vi "MessagingPlayground.vi"() -> ()   [LabVIEW 2019]
uses:
  <userlib>/LevyLab/Instrument Framework/SMOs/RemoteControl/Typedefs/RC Com Type--enum.ctl
  <userlib>/LevyLab/Instrument Framework/SMOs/RemoteControl/RemoteControl.lvclass
  C:/Program Files (x86)/National Instruments/LabVIEW 2019/vi.lib/JKI/JKI SMO/SMO/SMO.lvclass
  <vilib>/JKI/JKI SMO/SMO/SMO.lvclass
panel:
  out "IDs":string[](array[string])
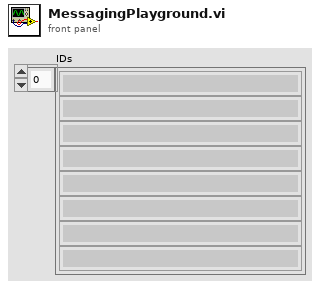
[diagram p1: front panel]
types:
  T1 = typedef "RemoteControl.lvclass/RC Com Type--enum.ctl" = enum16{"RC", "STM", "ZMQ"}
  T2 = enum32{"Invalid", "Standard", "Closed", "Hidden", "Minimized", "Maximized"}
  T3 = enum32{"invalid app kind", "Development System", "Run Time System", "Student Edition", "Embedded LabVIEW", "Evaluation", "Custom"}
  T4 = cluster{"Core":cluster{"Current VI Reference":refnum<vi>, "Close Panel on Exit?":bool}, "RC":refnum<class "RemoteControl.lvclass">, "IDs":string[]}
  T5 = cluster{"Current VI Reference":refnum<vi>, "Close Panel on Exit?":bool}
  T6 = typedef "RemoteControl.lvclass/PublicEvents--Cluster.ctl" = cluster{"SendMessageFromProcess":refnum<user-event>}
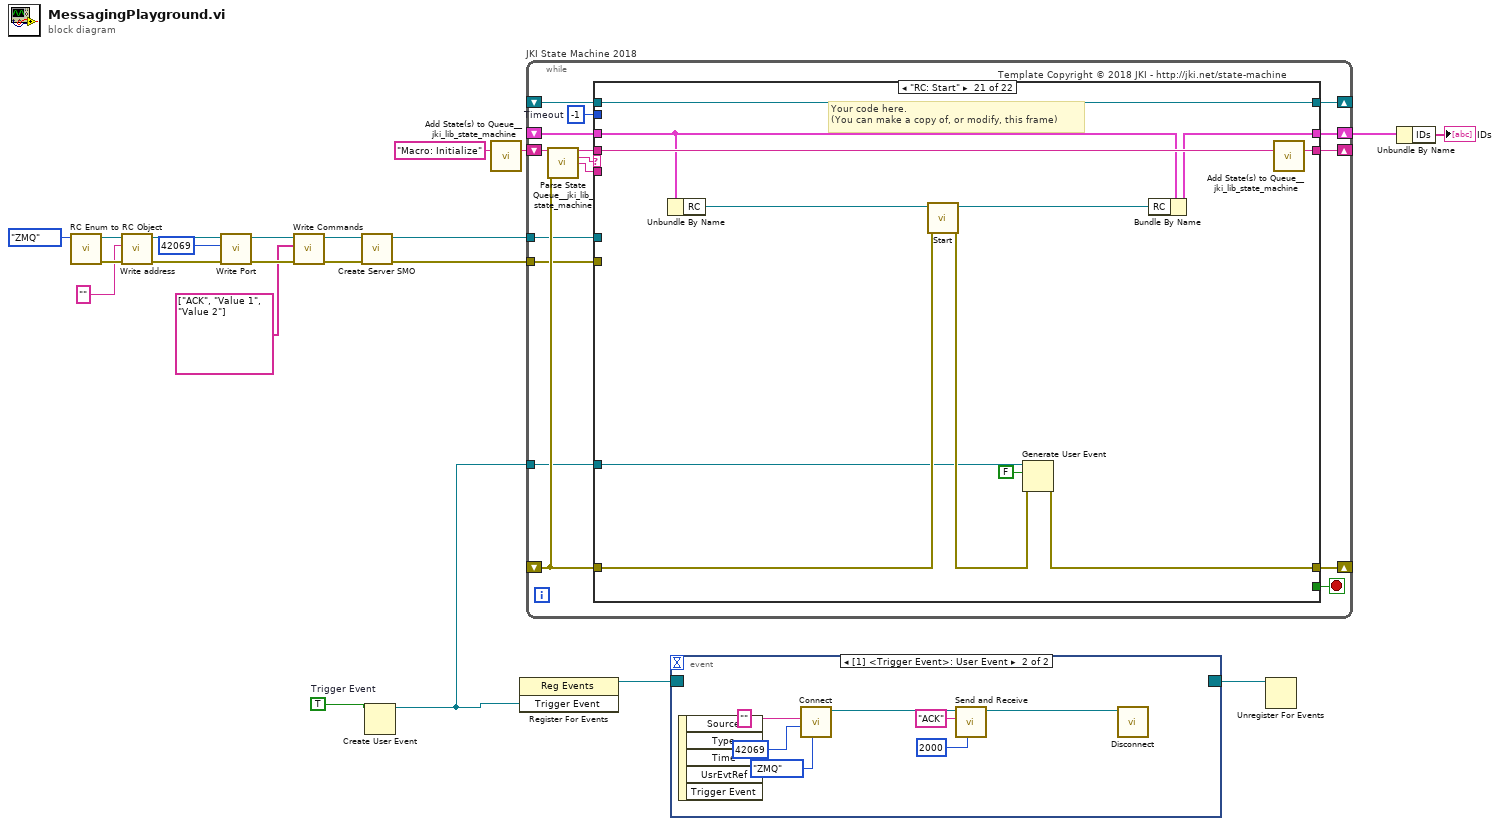
[diagram p0: block diagram]
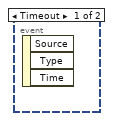
[diagram p2: hidden frame]
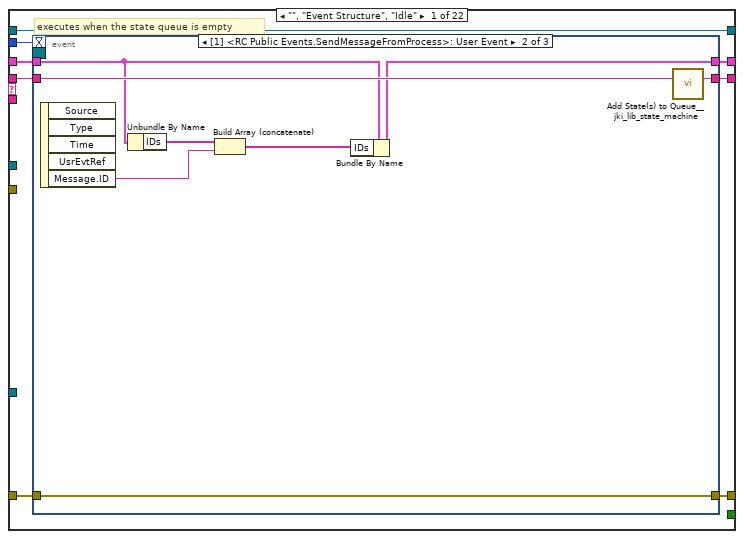
[diagram p3: hidden frame]
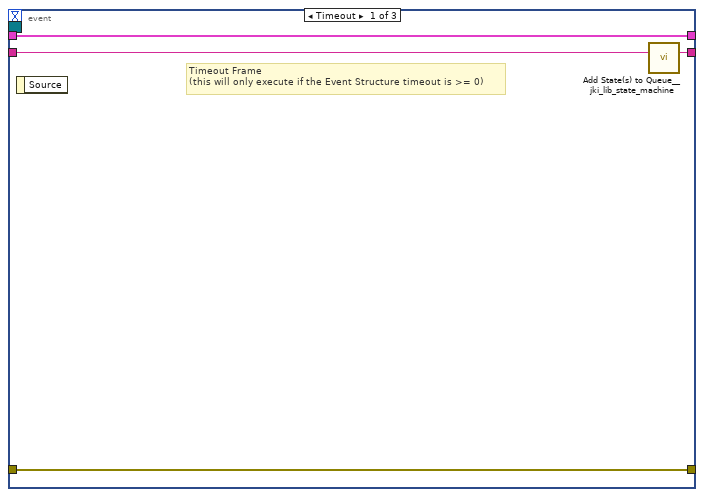
[diagram p4: hidden frame]
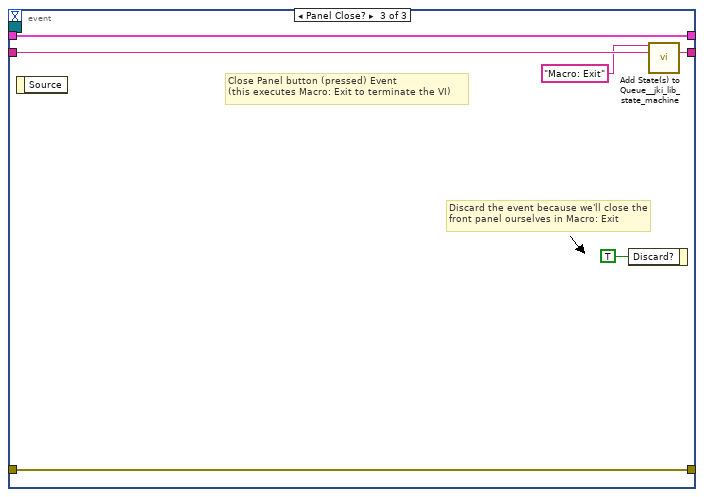
[diagram p5: hidden frame]
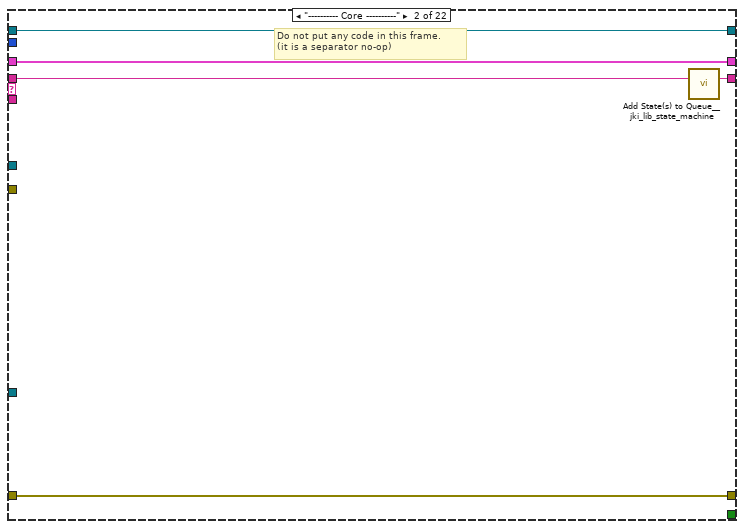
[diagram p6: hidden frame]
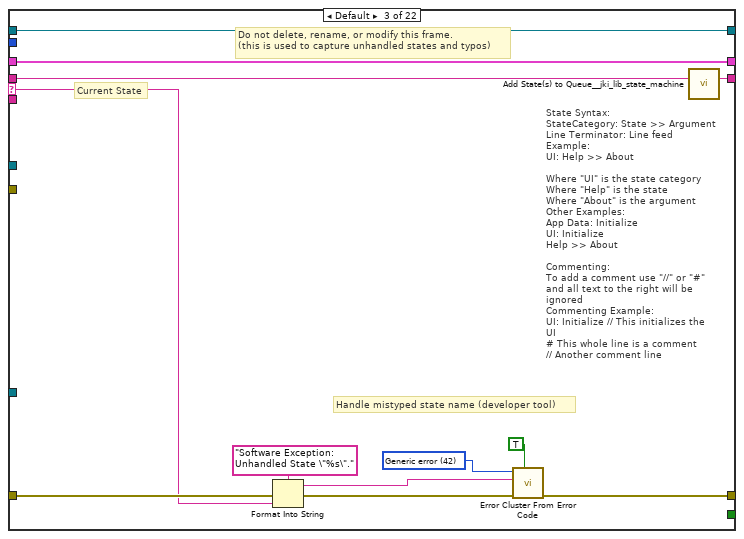
[diagram p7: hidden frame]
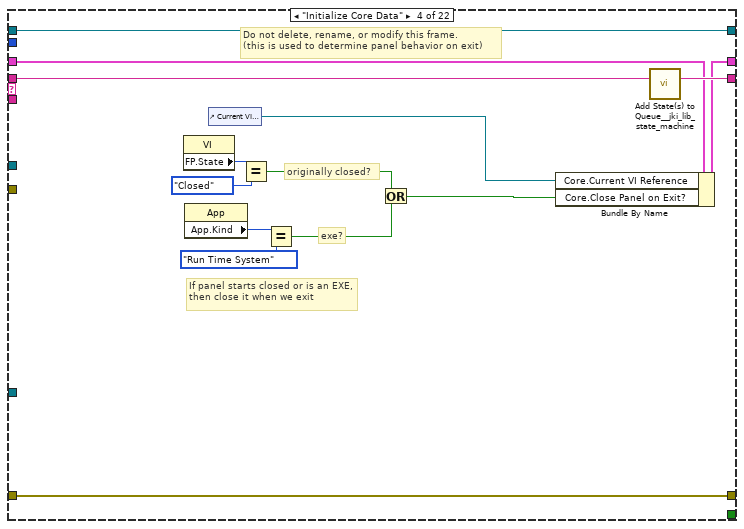
[diagram p8: hidden frame]
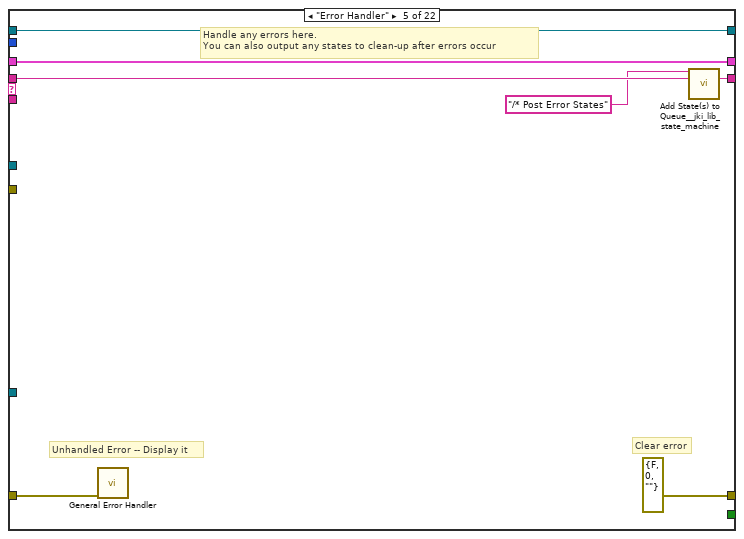
[diagram p9: hidden frame]
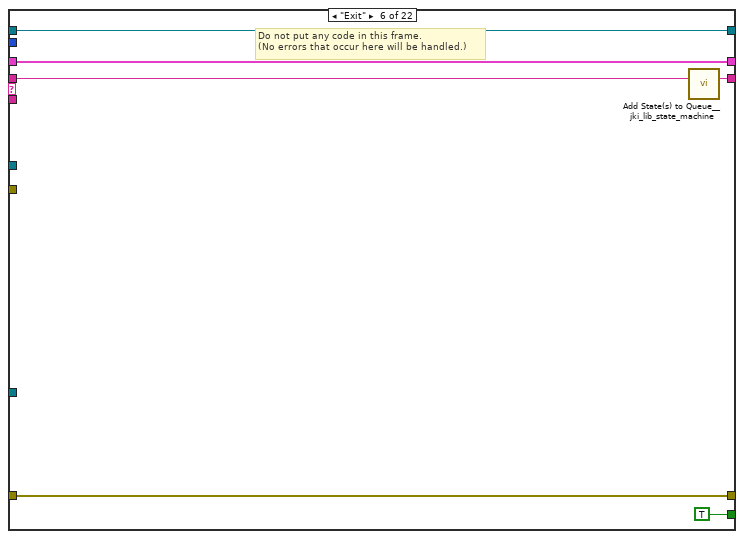
[diagram p10: hidden frame]
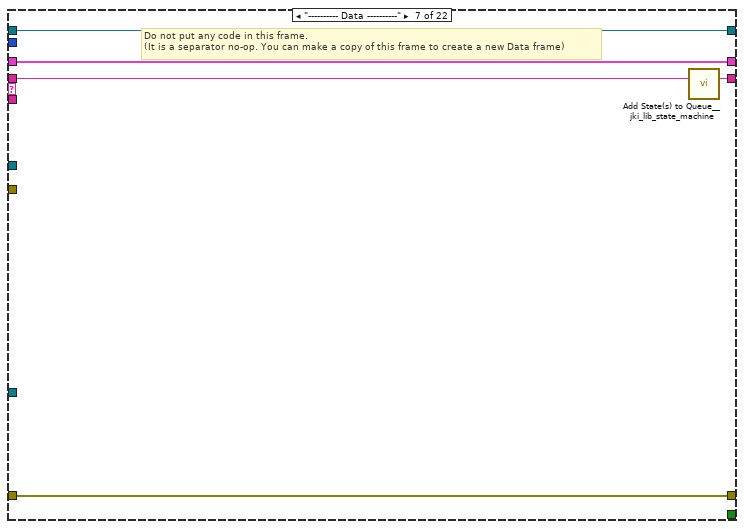
[diagram p11: hidden frame]
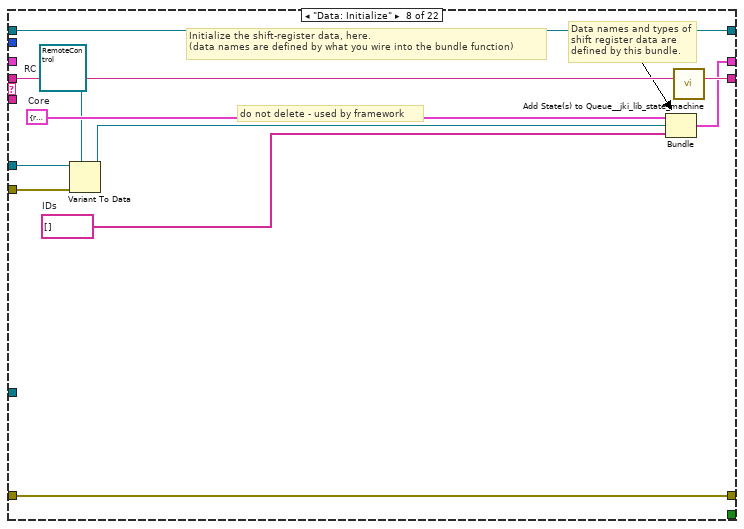
[diagram p12: hidden frame]
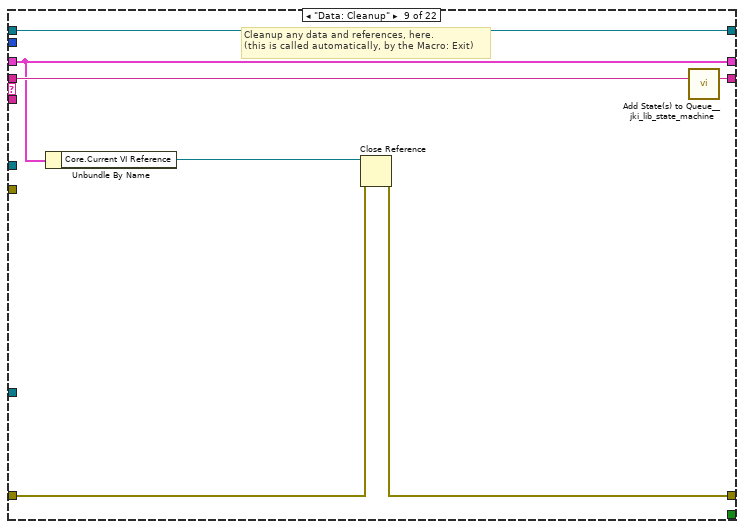
[diagram p13: hidden frame]
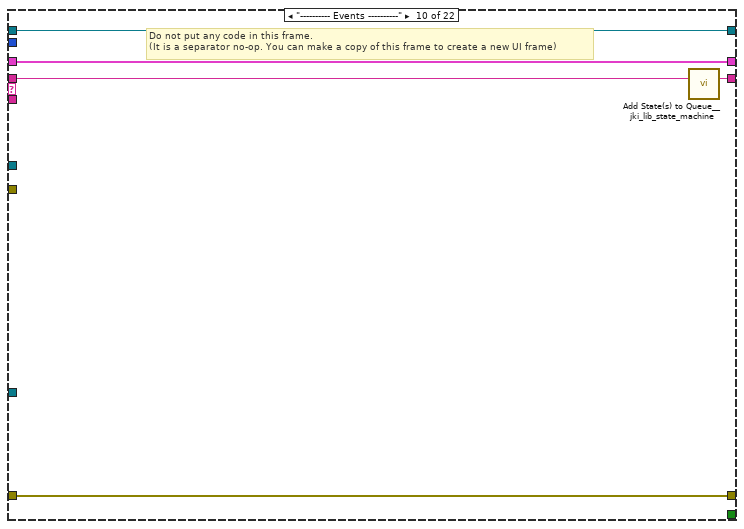
[diagram p14: hidden frame]
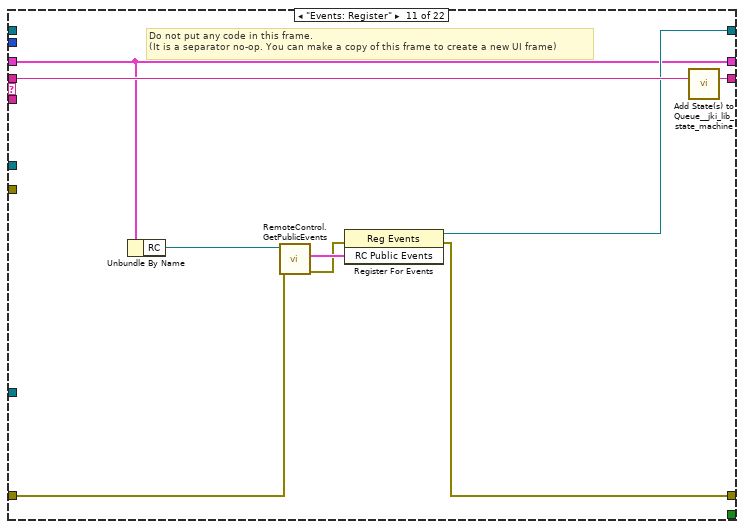
[diagram p15: hidden frame]
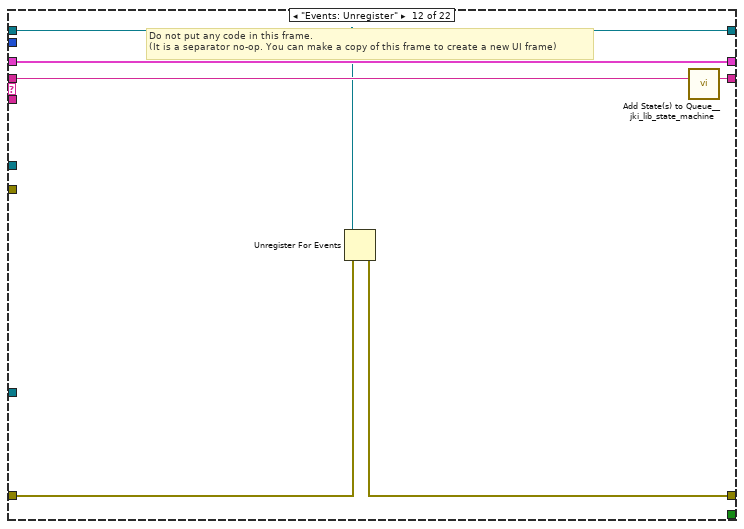
[diagram p16: hidden frame]
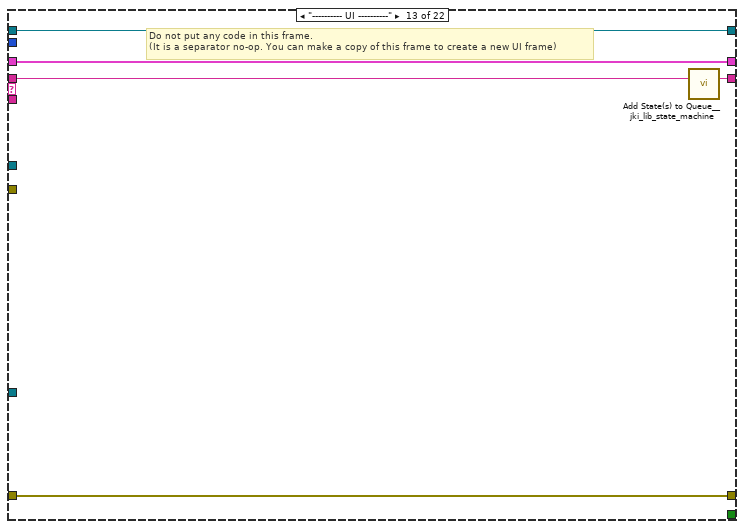
[diagram p17: hidden frame]
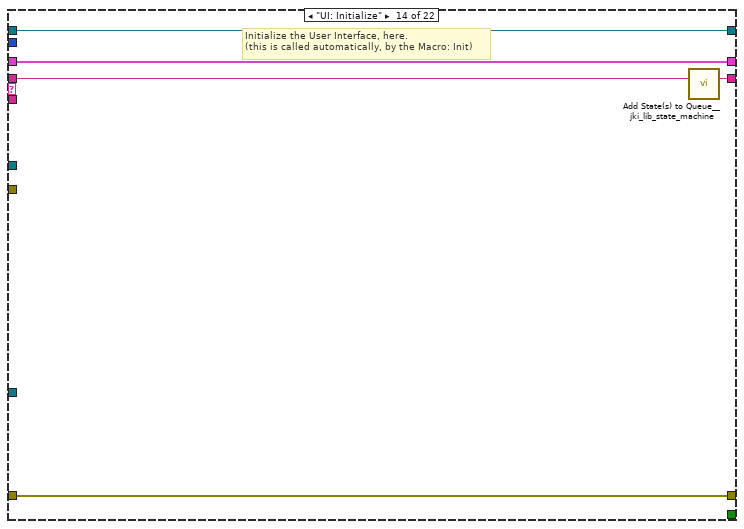
[diagram p18: hidden frame]
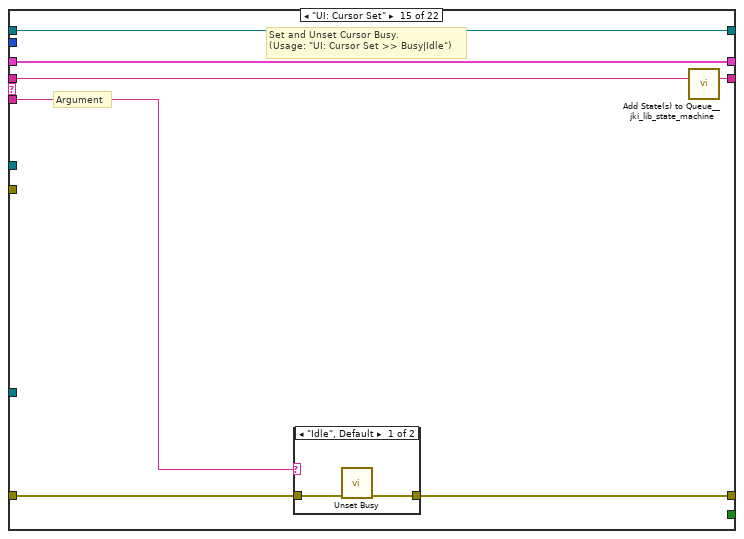
[diagram p19: hidden frame]
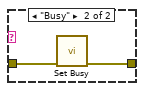
[diagram p20: hidden frame]
diagram:
  w6 = TRUE  # Trigger Event
  n1 = call <userlib>:"RC Enum to RC Object.vi"("RC Type"=RC_Com_Type--enum."ZMQ") -> ("error out"=w17:errorcluster, "RemoteControl out"=w18:refnum<class "RemoteControl.lvclass">)  [unwired: 9 in]
  n2 = call-dynamic "Write address.vi"("error in (no error)"=w17, "address"="", "RemoteControl in"=w18) -> ("error out"=w21:errorcluster, "RemoteControl out"=w22:refnum<class "RemoteControl.lvclass">)  [unwired: 7 in]
  n3 = call-dynamic "Write Port.vi"("error in (no error)"=w21, "Port"=u16 42069, "RemoteControl in"=w22) -> ("error out"=w19:errorcluster, "RemoteControl out"=w20:refnum<class "RemoteControl.lvclass">)  [unwired: 7 in]
  n4 = call-dynamic "Write Commands.vi"("error in (no error)"=w19, "Commands"=string[] ["ACK", "Value 1", "Value 2"], "RemoteControl in"=w20) -> ("error out"=w13:errorcluster, "RemoteControl out"=w14:refnum<class "RemoteControl.lvclass">)  [unwired: 7 in]
  n5 = call-dynamic "Create Server SMO.vi"("error in (no error)"=w13, "RemoteControl in"=w14) -> ("error out"=w9:errorcluster, "RemoteControl out"=w10:refnum<class "RemoteControl.lvclass">)  [unwired: 8 in]
  n6 = Create User Event(user event datatype=w6) -> (user event=w4:refnum<user-event>)  [unwired: 1 in, 1 out]
  n7 = call <vilib>:"Add State(s) to Queue__jki_lib_state_machine.vi"("State(s) in (\"\")"="Macro: Initialize") -> ("States Out"=w12:string)  [unwired: 14 in]
  n8 = register-events(w4) -> (reference out=w5:refnum<event-registration>)  [unwired: 2 in, 1 out]
  n9 = while "JKI State Machine 2018" {
    shift-right: [w31] -> w2
    shift-left: _ -> [w30]
    shift-right: [w34] -> _
    shift-left: _ -> [w28]
    shift-right: [w33] -> _
    shift-left: w12 -> [w35]
    tunnel: w10 -> [w27]
    tunnel: w9 -> [w26]
    shift-right: [w25] -> _
    shift-left: _ -> [w24]
    tunnel: w4 -> [w23]
    stop <- w32 stop-if-true
    w29 = -1  # Timeout
    # "Template Copyright © 2018 JKI - http://jki.net/state-machine"
    n10 = call <vilib>:"Parse State Queue__jki_lib_state_machine.vi"("State Queue"=w35, "Error In (no error)"=w28) -> ("Remaining States"=w37:string, "Current State"=w38:string, "Arguments"=w36:string)  [unwired: 11 in]
    n11 = case shown="\"RC: Start\"" w38 {
      selector: w38 -> [_ _ w71 _ _ _ _ _ _ _ _ _ _ _ _ _ _ _ _ _ _ _]
      tunnel: w37 -> [w46 w69 w75 w95 w102 w108 w113 w124 w131 w136 w145 w151 w156 w161 w168 w180 w250 w256 w267 w272 w284 w295]
      tunnel: w36 -> [_ _ _ _ _ _ _ _ _ _ _ _ _ _ w163 w174 _ _ _ _ _ _]
      tunnel: w30 -> [w44 w66 w73 w88 w99 w106 w110 _ w126 w133 w141 w149 w153 w159 w166 w176 w247 w253 w264 w269 w281 w292]
      tunnel: [w43 w67 w77 w92 errorcluster {"status"=FALSE, "code"=0, "source"=""} ("error out") w105 w111 w121 w127 w134 w142 w146 w154 w158 w164 w177 w248 w254 w265 w270 w275 w287] -> w34
      tunnel: w28 -> [w42 w67 w76 w92 w98 w105 w111 w121 w128 w134 w137 w147 w154 w158 w165 w178 w248 w254 w265 w270 w278 w286]
      tunnel: [w45 w68 w74 w94 w101 w107 w112 w123 w130 w135 w144 w150 w155 w160 w167 w179 w249 w255 w266 w271 w283 w294] -> w33
      tunnel: [_ _ _ _ _ TRUE _ _ _ _ _ _ _ _ _ _ _ _ _ _ _ _] -> w32
      tunnel: [w41 w66 w73 w93 w99 w106 w110 w122 w126 w133 w141 w149 w153 w159 w166 w176 w247 w253 w264 w269 w282 w293] -> w31
      tunnel: w29 -> [w40 _ _ _ _ _ _ _ _ _ _ _ _ _ _ _ _ _ _ _ _ _]
      tunnel: w27 -> [_ _ _ _ _ _ _ w119 _ _ _ _ _ _ _ _ _ _ _ _ _ _]
      tunnel: w26 -> [_ _ _ _ _ _ _ w116 _ _ _ _ _ _ _ _ _ _ _ _ _ _]
      tunnel: [w39 w65 w70 w82 w96 w103 w109 w115 w125 w132 w143 w148 w152 w157 w162 w173 w246 w251 w257 w268 w277 w285] -> w25
      tunnel: w24 -> [w39 w65 w70 w82 w96 w103 w109 w115 w125 w132 _ w148 w152 w157 w162 w173 w246 w251 w257 w268 w277 w285]
      tunnel: w23 -> [_ _ _ _ _ _ _ _ _ _ _ _ _ _ _ _ _ _ _ _ w274 _]
      frame "", "Event Structure", "Idle" {
        # "executes when the state queue is empty"
        n12 = event shown="[1] <RC Public Events.SendMessageFromProcess>: User Event" {
          selector: w39 -> [_ _ _]
          dyn-events: _ -> [_ _ _]
          timeout: w40 -> [_ _ _]
          tunnel: w46 -> [w50 w58 w64]
          tunnel: [w49 w57 w63] -> w45
          tunnel: w44 -> [w47 w54 w61]
          tunnel: [w48 w56 w62] -> w43
          tunnel: w42 -> [w48 w56 w62]
          tunnel: [w47 w55 w61] -> w41
          event Timeout {
            # "Timeout Frame\n(this will only execute if the Event Structure timeout is >= 0)"
            n13 = event-data() -> ()  [unwired: 1 in, 1 out]
            n14 = call <vilib>:"Add State(s) to Queue__jki_lib_state_machine.vi"("State(s) in (\"\")"=w50) -> ("States Out"=w49:string)  [unwired: 14 in]
          }
          event User Event {
            n15 = event-data() -> ("Message.ID"=w52:string)  [unwired: 1 in, 4 out]
            n16 = Unbundle By Name(w54) -> ("IDs"=w53:string[])
            n17 = Build Array (concatenate)(w53, w52) -> (w51:string[])
            n18 = Bundle By Name(cluster=w54, "IDs"=w51) -> (w55:T4)
            n19 = call <vilib>:"Add State(s) to Queue__jki_lib_state_machine.vi"("State(s) in (\"\")"=w58) -> ("States Out"=w57:string)  [unwired: 14 in]
          }
          event Panel Close? {
            # "Discard the event because we'll close the front panel ourselves in Macro: Exit"
            # "Close Panel button (pressed) Event\n(this executes Macro: Exit to terminate the VI)"
            n20 = event-data() -> ()  [unwired: 1 in, 1 out]
            n21 = event-data("Discard?"=TRUE) -> ()  [unwired: 1 in, 1 out]
            n22 = call <vilib>:"Add State(s) to Queue__jki_lib_state_machine.vi"("State(s) in Front (\"\")"="Macro: Exit", "State(s) in (\"\")"=w64) -> ("States Out"=w63:string)  [unwired: 13 in]
          }
        }
      }
      frame "---------- Core ----------" {
        # "Do not put any code in this frame.\n(it is a separator no-op)"
        n23 = call <vilib>:"Add State(s) to Queue__jki_lib_state_machine.vi"("State(s) in (\"\")"=w69) -> ("States Out"=w68:string)  [unwired: 14 in]
      }
      frame Default {
        w80 = 42 items=["No error", "Argument error", "Memory is full", "Out of zone", "End of file", "File already open", "Generic file I/O error", "File not found", "File permission error", "Disk is full", "Duplicate path", "Too many files open", "System feature not enabled", "Resource file not found", "Cannot add resource", "Resource not found", "Image not found", "Image memory error", "Pen does not exist", "Config type invalid", "Config token not found", "Config parse error", "Config memory error", "Bad external code format", "Bad external code offset", "External code not present", "Null window", "Destroy window error", "Null menu", "Print aborted", "Bad print record", "Print driver error", "Windows error during printing", "Memory error during printing", "Print dialog error", "Generic print error", "Invalid device refnum", "Device not found", "Device parameter error", "Device unit error", "Cannot open device", "Device call aborted", "Generic error", "Cancelled by user", "Object ID too low", "Object ID too high", "Object not in heap", "Unknown heap", "Unknown object (invalid DefProc)", "Unknown object (DefProc not in table)", "Message out of range", "Invalid (null) method", "Unknown message", "Manager call not supported", "Bad address", "Network operation in progress", "Network operation timed out", "Connection is busy", "Network attribute not supported", "Network error", "Address in use", "System out of memory", "Connection aborted", "Connection refused", "Not connected", "Already connected", "Connection closed", "Initialization error (interapplication manager)", "Bad occurrence", "Wait on unbound occurrence handler", "Occurrence queue overflow", "Datalog type conflict", "Unused", "Unrecognized type (interapplication manager)", "Memory corrupt", "Failed to make temporary DLL", "Old CIN version", "Drag socket not found", "Failed to load drop-object", "Failed to register OLE object", "Failed to release OLE object", "Format specifier type mismatch", "Unknown format specifier", "Too few format specifiers", "Too many format specifiers", "Scan failed", "Newer CIN version", "Error converting to variant", "Runtime menu error", "Password tampered", "Variant attribute not found", "Incompatible variant data type", "Event data is not available", "Event Store is not present", "Occurrence is not found", "Event Queue is not created", "Event info is not available", "Refnum passed is NULL", "Error retrieving Class GUID", "Error retrieving CoClass GUID", "Error retrieving TypeLib GUID.", "Bad built application magic bytes.", "Specific driver is different from the specific driver associated with the Logical Name.", "There is no session opened to the class driver.", "Max Error", "MAX - Error with config objects", "MAX - Error loading configuration", "MAX - Group not supported"]
        # "State Syntax:\nStateCategory: State >> Argument\nLine Terminator: Line feed\nExample:\nUI: Help >> About\n\nWhere \"UI\" is the state category\nWhere \"Help\" is the state\nWhere \"About\" is the argument\nOther Examples:\nApp Data: Initialize\nUI: Initialize\nHelp >> About\n\nCommenting:\nTo add a comment use \"//\" or \"#\" and all text to the right will be ignored\nCommenting Example:\nUI: Initialize // This initializes the UI\n# This whole line is a comment\n// Another comment line"
        # "Current State"
        # "Do not delete, rename, or modify this frame.\n(this is used to capture unhandled states and typos)"
        # "Handle mistyped state name (developer tool)"
        n24 = Format Into String(format string="Software Exception: Unhandled State \"%s\"." ("message"), error in=w76, w71) -> (resulting string=w79:string, error out=w78:errorcluster)  [unwired: 1 in]
        n25 = call <vilib>:"Error Cluster From Error Code.vi"("show call chain? (False)"=TRUE, "error in (no error)"=w78, "error message (\"\")"=w79, "error code (0)"=w80) -> ("error out"=w77:errorcluster)  [unwired: 5 in]
        n26 = call <vilib>:"Add State(s) to Queue__jki_lib_state_machine.vi"("State(s) in (\"\")"=w75) -> ("States Out"=w74:string)  [unwired: 14 in]
      }
      frame "Initialize Core Data" {
        # "Do not delete, rename, or modify this frame.\n(this is used to determine panel behavior on exit)"
        # "originally closed?"
        # "exe?"
        # "If panel starts closed or is an EXE, then close it when we exit"
        n27 = property class="VI"() -> ("FP.State"=w85:T2)  [unwired: 2 in, 2 out]
        n28 = property class="App"() -> ("App.Kind"=w91:T3)  [unwired: 2 in, 2 out]
        n29 = control-ref of="Current VI Reference"() -> (w86:refnum<vi>)
        n30 = Equal?(x=w85, y=T2."Closed" ("Front Panel Window:State")) -> (x = y?=w83:bool)
        n31 = Equal?(x=w91, y=T3."Run Time System" ("Application:Kind")) -> (x = y?=w89:bool)
        n32 = Or(x=w83, y=w89) -> (x .or. y?=w87:bool)
        n33 = Bundle By Name(cluster=w88, "Core.Current VI Reference"=w86, "Core.Close Panel on Exit?"=w87) -> (w93:T4)
        n34 = call <vilib>:"Add State(s) to Queue__jki_lib_state_machine.vi"("State(s) in (\"\")"=w95) -> ("States Out"=w94:string)  [unwired: 14 in]
      }
      frame "Error Handler" {
        # "Unhandled Error -- Display it"
        # "Handle any errors here.\nYou can also output any states to clean-up after errors occur"
        # "Clear error"
        n35 = call <vilib>:"General Error Handler.vi"("error in (no error)"=w98) -> ()  [unwired: 10 in, 5 out]
        n36 = call <vilib>:"Add State(s) to Queue__jki_lib_state_machine.vi"("State(s) in Front (\"\")"="/* Post Error States", "State(s) in (\"\")"=w102) -> ("States Out"=w101:string)  [unwired: 13 in]
      }
      frame "Exit" {
        # "Do not put any code in this frame.\n(No errors that occur here will be handled.)"
        n37 = call <vilib>:"Add State(s) to Queue__jki_lib_state_machine.vi"("State(s) in (\"\")"=w108) -> ("States Out"=w107:string)  [unwired: 14 in]
      }
      frame "---------- Data ----------" {
        # "Do not put any code in this frame.\n(It is a separator no-op. You can make a copy of this frame to create a new Data frame)"
        n38 = call <vilib>:"Add State(s) to Queue__jki_lib_state_machine.vi"("State(s) in (\"\")"=w113) -> ("States Out"=w112:string)  [unwired: 14 in]
      }
      frame "Data: Initialize" {
        w114 = string[] []  # IDs
        w118 = refnum<class "RemoteControl.lvclass"> refnum  # RC
        w120 = T5 {"Current VI Reference"=refnum, "Close Panel on Exit?"=FALSE}  # Core
        # "do not delete - used by framework"
        # "Data names and types of shift register data are defined by this bundle."
        # "Initialize the shift-register data, here.\n(data names are defined by what you wire into the bundle function)"
        n39 = Variant To Data(error in=w116, type=w118, Variant=w119) -> (data=w117:refnum<class "RemoteControl.lvclass">)  [unwired: 1 out]
        n40 = Bundle("Core"=w120, "RC"=w117, "IDs"=w114) -> (w122:T4)  [unwired: 1 in]
        n41 = call <vilib>:"Add State(s) to Queue__jki_lib_state_machine.vi"("State(s) in (\"\")"=w124) -> ("States Out"=w123:string)  [unwired: 14 in]
      }
      frame "Data: Cleanup" {
        # "Cleanup any data and references, here.\n(this is called automatically, by the Macro: Exit)"
        n42 = Unbundle By Name(w126) -> ("Core.Current VI Reference"=w129:refnum<vi>)
        n43 = Close Reference(reference=w129, error in (no error)=w128) -> (error out=w127:errorcluster)
        n44 = call <vilib>:"Add State(s) to Queue__jki_lib_state_machine.vi"("State(s) in (\"\")"=w131) -> ("States Out"=w130:string)  [unwired: 14 in]
      }
      frame "---------- Events ----------" {
        # "Do not put any code in this frame.\n(It is a separator no-op. You can make a copy of this frame to create a new UI frame)"
        n45 = call <vilib>:"Add State(s) to Queue__jki_lib_state_machine.vi"("State(s) in (\"\")"=w136) -> ("States Out"=w135:string)  [unwired: 14 in]
      }
      frame "Events: Register" {
        # "Do not put any code in this frame.\n(It is a separator no-op. You can make a copy of this frame to create a new UI frame)"
        n46 = Unbundle By Name(w141) -> ("RC"=w140:refnum<class "RemoteControl.lvclass">)
        n47 = call <userlib>:"RemoteControl.GetPublicEvents.vi"("error in (no error)"=w137, "RemoteControl"=w140) -> ("error out"=w138:errorcluster, "RC Public Events"=w139:T6)  [unwired: 7 in, 1 out]
        n48 = register-events(error in=w138, w139) -> (reference out=w143:refnum<event-registration>, error out=w142:errorcluster)  [unwired: 1 in]
        n49 = call <vilib>:"Add State(s) to Queue__jki_lib_state_machine.vi"("State(s) in (\"\")"=w145) -> ("States Out"=w144:string)  [unwired: 14 in]
      }
      frame "Events: Unregister" {
        # "Do not put any code in this frame.\n(It is a separator no-op. You can make a copy of this frame to create a new UI frame)"
        n50 = Unregister For Events(event registration refnum=w148, error in=w147) -> (error out=w146:errorcluster)
        n51 = call <vilib>:"Add State(s) to Queue__jki_lib_state_machine.vi"("State(s) in (\"\")"=w151) -> ("States Out"=w150:string)  [unwired: 14 in]
      }
      frame "---------- UI ----------" {
        # "Do not put any code in this frame.\n(It is a separator no-op. You can make a copy of this frame to create a new UI frame)"
        n52 = call <vilib>:"Add State(s) to Queue__jki_lib_state_machine.vi"("State(s) in (\"\")"=w156) -> ("States Out"=w155:string)  [unwired: 14 in]
      }
      frame "UI: Initialize" {
        # "Initialize the User Interface, here.\n(this is called automatically, by the Macro: Init)"
        n53 = call <vilib>:"Add State(s) to Queue__jki_lib_state_machine.vi"("State(s) in (\"\")"=w161) -> ("States Out"=w160:string)  [unwired: 14 in]
      }
      frame "UI: Cursor Set" {
        # "Argument"
        # "Set and Unset Cursor Busy.\n(Usage: \"UI: Cursor Set >> Busy|Idle\")"
        n54 = case shown="\"Idle\", Default" w163 {
          tunnel: w165 -> [w170 w172]
          tunnel: [w169 w171] -> w164
          frame "Idle", Default {
            n55 = call <vilib>:"Unset Busy.vi"("error in (no error)"=w170) -> ("error out"=w169:errorcluster)  [unwired: 10 in]
          }
          frame "Busy" {
            n56 = call <vilib>:"Set Busy.vi"("error in (no error)"=w172) -> ("error out"=w171:errorcluster)  [unwired: 9 in, 1 out]
          }
        }
        n57 = call <vilib>:"Add State(s) to Queue__jki_lib_state_machine.vi"("State(s) in (\"\")"=w168) -> ("States Out"=w167:string)  [unwired: 14 in]
      }
      frame "UI: Front Panel State" {
        # "Argument"
        # "Set Front Panel Open or Closed\n(Usage: \"UI: Front Panel State >> Open|Close\")"
        n58 = Unbundle By Name(w176) -> ("Core.Current VI Reference"=w175:refnum<vi>)
        n59 = case shown="\"Minimize\", \"Minimized\"" w174 {
          tunnel: w178 -> [w186 w201 w212 w225 w238]
          tunnel: [w188 w202 w214 w227 w240] -> w177
          tunnel: w175 -> [w187 w199 w213 w226 w239]
          frame "Open", "Standard", Default {
            w181 = T2."Standard" ("State")
            n60 = property class="VI"(reference=w187, error in=w186) -> (reference out=w184:refnum<vi>, error out=w185:errorcluster, "FP.State"=w183:T2)
            n61 = Not Equal?(x=w183, y=w181) -> (x != y?=w182:bool)
            n62 = case shown="True" w182 {
              tunnel: [w192 w194] -> w188
              tunnel: w185 -> [w191 w194]
              tunnel: w184 -> [w190 _]
              tunnel: w181 -> [w189 _]
              frame True {
                n63 = invoke class="VI" method="FP.Open"(reference=w190, error in=w191, "Activate"=TRUE, "State"=w189) -> (error out=w192:errorcluster)  [unwired: 1 in, 4 out]
              }
              frame False {
              }
            }
          }
          frame "Close", "Closed" {
            n64 = property class="VI"(reference=w199, error in=w201) -> (reference out=w198:refnum<vi>, error out=w200:errorcluster, "FP.State"=w196:T2)
            n65 = Not Equal?(x=w196, y=T2."Closed" ("Front Panel Window:State")) -> (x != y?=w195:bool)
            n66 = case shown="True" w195 {
              tunnel: [w203 w206] -> w202
              tunnel: w200 -> [w203 w205]
              tunnel: w198 -> [_ w204]
              frame False {
              }
              frame True {
                n67 = invoke class="VI" method="FP.Close"(reference=w204, error in=w205) -> (error out=w206:errorcluster)  [unwired: 1 in, 2 out]
              }
            }
          }
          frame "Hidden", "Hide" {
            w207 = T2."Hidden" ("State")
            n68 = property class="VI"(reference=w213, error in=w212) -> (reference out=w210:refnum<vi>, error out=w211:errorcluster, "FP.State"=w209:T2)
            n69 = Not Equal?(x=w209, y=w207) -> (x != y?=w208:bool)
            n70 = case shown="True" w208 {
              tunnel: [w218 w219] -> w214
              tunnel: w211 -> [w217 w219]
              tunnel: w210 -> [w216 _]
              tunnel: w207 -> [w215 _]
              frame True {
                n71 = invoke class="VI" method="FP.Open"(reference=w216, error in=w217, "State"=w215) -> (error out=w218:errorcluster)  [unwired: 2 in, 4 out]
              }
              frame False {
              }
            }
          }
          frame "Minimize", "Minimized" {
            w220 = T2."Minimized" ("State")
            n72 = property class="VI"(reference=w226, error in=w225) -> (reference out=w223:refnum<vi>, error out=w224:errorcluster, "FP.State"=w222:T2)
            n73 = Not Equal?(x=w222, y=w220) -> (x != y?=w221:bool)
            n74 = case shown="True" w221 {
              tunnel: [w231 w232] -> w227
              tunnel: w224 -> [w230 w232]
              tunnel: w223 -> [w229 _]
              tunnel: w220 -> [w228 _]
              frame True {
                n75 = invoke class="VI" method="FP.Open"(reference=w229, error in=w230, "State"=w228) -> (error out=w231:errorcluster)  [unwired: 2 in, 4 out]
              }
              frame False {
              }
            }
          }
          frame "Maximize", "Maximized" {
            w233 = T2."Maximized" ("State")
            n76 = property class="VI"(reference=w239, error in=w238) -> (reference out=w236:refnum<vi>, error out=w237:errorcluster, "FP.State"=w235:T2)
            n77 = Not Equal?(x=w235, y=w233) -> (x != y?=w234:bool)
            n78 = case shown="True" w234 {
              tunnel: [w244 w245] -> w240
              tunnel: w237 -> [w243 w245]
              tunnel: w236 -> [w242 _]
              tunnel: w233 -> [w241 _]
              frame True {
                n79 = invoke class="VI" method="FP.Open"(reference=w242, error in=w243, "State"=w241) -> (error out=w244:errorcluster)  [unwired: 2 in, 4 out]
              }
              frame False {
              }
            }
          }
        }
        n80 = call <vilib>:"Add State(s) to Queue__jki_lib_state_machine.vi"("State(s) in (\"\")"=w180) -> ("States Out"=w179:string)  [unwired: 14 in]
      }
      frame "---------- Macro ----------" {
        # "Do not put any code in this frame.\n(It is a separator no-op. You can make a copy of this frame to create a new Macro frame)"
        n81 = call <vilib>:"Add State(s) to Queue__jki_lib_state_machine.vi"("State(s) in (\"\")"=w250) -> ("States Out"=w249:string)  [unwired: 14 in]
      }
      frame "Macro: Initialize" {
        # "Initialization Macro\n(This is called once, when the VI starts)"
        n82 = call <vilib>:"Add State(s) to Queue__jki_lib_state_machine.vi"("State(s) in Front (\"\")"="Data: Initialize\nInitialize Core Data\nEvents: Register\nUI: Initialize\nUI: Front Panel State >> Open\nRC: Start", "State(s) in (\"\")"=w256) -> ("States Out"=w255:string)  [unwired: 13 in]
      }
      frame "Macro: Exit" {
        # "Exit Macro\n(This is called once, when the VI exits)"
        n83 = Unbundle By Name(w264) -> ("Core.Close Panel on Exit?"=w263:bool)
        n84 = Select(t="UI: Front Panel State >> Close", s=w263, f="") -> (s? t:f=w260:string)
        n85 = call <vilib>:"Add State(s) to Queue__jki_lib_state_machine.vi"("State(s) in (\"\")"=w260, "State(s) at Back (\"\")"="RC: Stop\nData: Cleanup\nEvents: Unregister\nExit") -> ("States Out"=w258:string)  [unwired: 13 in]
        n86 = call <vilib>:"Add State(s) to Queue__jki_lib_state_machine.vi"("State(s) in Front (\"\")"=w258, "State(s) in (\"\")"=w267) -> ("States Out"=w266:string)  [unwired: 13 in]
      }
      frame "---------- RC ----------" {
        # "Template Separator\n(You can make a copy of, or modify, this frame)"
        n87 = call <vilib>:"Add State(s) to Queue__jki_lib_state_machine.vi"("State(s) in (\"\")"=w272) -> ("States Out"=w271:string)  [unwired: 14 in]
      }
      frame "RC: Start" {
        # "Your code here.\n(You can make a copy of, or modify, this frame)"
        n88 = Unbundle By Name(w281) -> ("RC"=w280:refnum<class "RemoteControl.lvclass">)
        n89 = call <vilib>:"Start.vi"("error in (no error)"=w278, "SMO"=w280) -> ("error out"=w276:errorcluster, "SMO out"=w279:refnum<class "RemoteControl.lvclass">)  [unwired: 8 in]
        n90 = Generate User Event(user event=w274, event data cluster=FALSE ("event data"), error in=w276) -> (error out=w275:errorcluster)  [unwired: 1 in, 1 out]
        n91 = Bundle By Name(cluster=w281, "RC"=w279) -> (w282:T4)
        n92 = call <vilib>:"Add State(s) to Queue__jki_lib_state_machine.vi"("State(s) in (\"\")"=w284) -> ("States Out"=w283:string)  [unwired: 14 in]
      }
      frame "RC: Stop" {
        # "Your code here.\n(You can make a copy of, or modify, this frame)"
        n93 = Unbundle By Name(w292) -> ("RC"=w291:refnum<class "RemoteControl.lvclass">)
        n94 = call <vilib>:"Stop.vi"("error in (no error)"=w286, "SMO"=w291) -> ("error out"=w288:errorcluster, "SMO out"=w290:refnum<class "RemoteControl.lvclass">)  [unwired: 8 in]
        n95 = call <vilib>:"Destroy.vi"("error in (no error)"=w288, "SMO"=w290) -> ("error out"=w287:errorcluster)  [unwired: 9 in]
        n96 = Bundle By Name(cluster=w292, "RC"=refnum<class "RemoteControl.lvclass"> refnum) -> (w293:T4)
        n97 = call <vilib>:"Add State(s) to Queue__jki_lib_state_machine.vi"("State(s) in (\"\")"=w295) -> ("States Out"=w294:string)  [unwired: 14 in]
      }
    }
  }
  n98 = event shown="[1] <Trigger Event>: User Event" {
    selector: w5 -> [_ _]
    dyn-events: [_ _] -> w3
    timeout: _ -> [_ _]
    event Timeout {
      n99 = event-data() -> ()  [unwired: 1 in, 3 out]
    }
    event User Event {
      n100 = event-data() -> ()  [unwired: 1 in, 5 out]
      n101 = call <userlib>:"Connect.vi"("RC Type"=RC_Com_Type--enum."ZMQ", "Port"=u16 42069, "address"="") -> ("RemoteControl out"=w302:refnum<class "RemoteControl.lvclass">)  [unwired: 7 in, 1 out]
      n102 = call <userlib>:"Send and Receive.vi"("timeout (ms) [500]"=2000, "Command"="ACK", "RemoteControl in"=w302) -> ("RemoteControl out"=w298:refnum<class "RemoteControl.lvclass">)  [unwired: 5 in, 3 out]
      n103 = call <userlib>:"Disconnect.vi"("RemoteControl in"=w298) -> ()  [unwired: 9 in, 2 out]
    }
  }
  n104 = Unregister For Events(event registration refnum=w3) -> ()  [unwired: 1 in, 1 out]
  n105 = Unbundle By Name(w2) -> ("IDs"=→"IDs":string[])
